vi "xwav2wave.vi"(4 "xwave":T1={"attributes"=variant, "X"={"start"=1.0, "delta"=1.0, "units"="index", "dim"="au"}, "Y"={"data"=[], "units"="au"}}) -> (1 "waveform":waveform(dbl))   [LabVIEW 2015]
uses:
  xwav.ctl
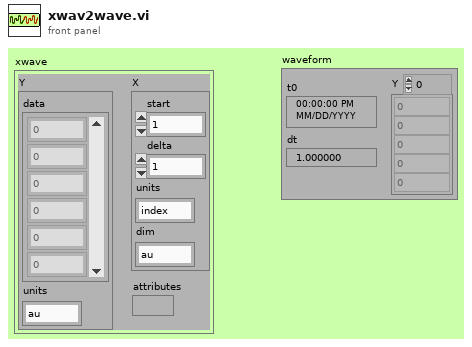
[diagram p1: front panel]
types:
  T1 = typedef "xwav.ctl" = cluster{"attributes":variant, "X":cluster{"start":dbl, "delta":dbl, "units":string, "dim":string}, "Y":cluster{"data":dbl[], "units":string}}
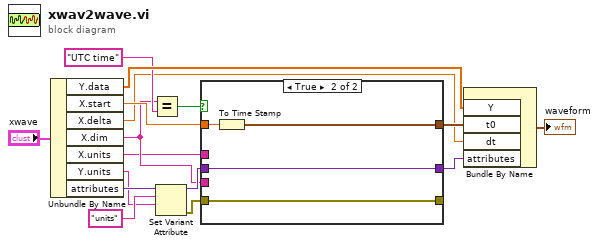
[diagram p0: block diagram]
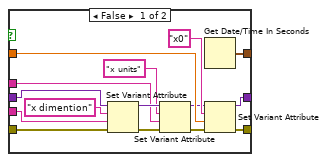
[diagram p2: hidden frame]
diagram:
  n1 = Unbundle By Name("xwave") -> ("Y.data"=w15:dbl[], "X.start"=w13:dbl, "X.delta"=w11:dbl, "X.dim"=w3:string, "X.units"=w1:string, "Y.units"=w6:string, "attributes"=w8:variant)
  n2 = Equal?(x=w3, y="UTC time" ("x units")) -> (x = y?=w9:bool)
  n3 = Set Variant Attribute(Variant=w8, name="units", value=w6) -> (Variant out=w5:variant, error out=w2:errorcluster)  [unwired: 1 in, 1 out]
  n4 = case shown="True" w9 {
    tunnel: w13 -> [w28 w35]
    tunnel: [w31 w34] -> w12
    tunnel: [w30 w33] -> w4
    tunnel: w5 -> [w27 w33]
    tunnel: w3 -> [w24 _]
    tunnel: w2 -> [w22 w32]
    tunnel: w1 -> [w20 _]
    tunnel: [w17 w32] -> _
    frame False {
      n5 = Set Variant Attribute(Variant=w27, name="x dimention", value=w24, error in=w22) -> (Variant out=w26:variant, error out=w19:errorcluster)  [unwired: 1 out]
      n6 = Set Variant Attribute(Variant=w26, name="x units", value=w20, error in=w19) -> (Variant out=w25:variant, error out=w18:errorcluster)  [unwired: 1 out]
      n7 = Get Date/Time In Seconds() -> (seconds since 1Jan1904=w31:timestamp)
      n8 = Set Variant Attribute(Variant=w25, name="x0", value=w28, error in=w18) -> (Variant out=w30:variant, error out=w17:errorcluster)  [unwired: 1 out]
    }
    frame True {
      n9 = To Time Stamp(1:w35) -> (0:w34:timestamp)
    }
  }
  n10 = Bundle By Name("Y"=w15, "t0"=w12, "dt"=w11, "attributes"=w4) -> (→"waveform":waveform(dbl))  [unwired: 1 in]
